vi "GetParameterValueBoolean.vi"(8 "error in (no error)":errorcluster, 11 "Parameter in":refnum<class "Parameter.lvclass">) -> (0 "error out":errorcluster, 2 "Value":bool, 3 "Parameter out":refnum<class "Parameter.lvclass">)   [LabVIEW 2023, in "Easy.SequenceManagerLabVIEW.lvlib" / "Parameter.lvclass"]
uses:
  Parameter.lvclass
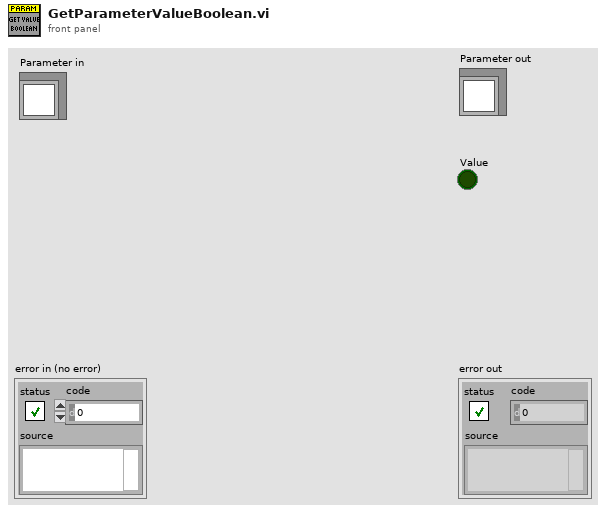
[diagram p1: front panel]
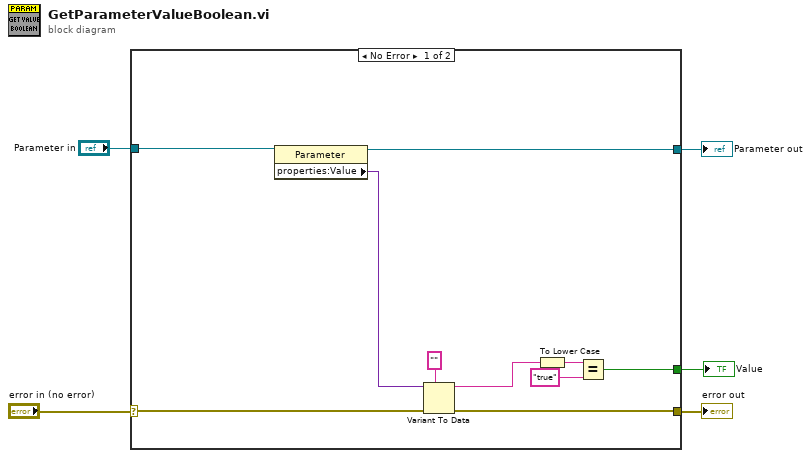
[diagram p0: block diagram]
diagram:
  n1 = case shown="No Error" "error in (no error)" {
    selector: "error in (no error)" -> [w15 w17]
    tunnel: [w12 w17] -> w4
    tunnel: "Parameter in" -> [w10 w16]
    tunnel: [w11 w16] -> w2
    tunnel: [w6 _] -> w1
    frame No Error {
      n2 = property class="Parameter"(reference=w10) -> (reference out=w11:refnum<class "Parameter.lvclass">, "properties:Value"=w13:variant)  [unwired: 1 in, 1 out]
      n3 = Variant To Data(error in=w15, type="", Variant=w13) -> (data=w9:string, error out=w12:errorcluster)
      n4 = To Lower Case(string=w9) -> (all lower case string=w8:string)
      n5 = Equal?(x=w8, y="true") -> (x = y?=w6:bool)
    }
    frame Error {
    }
  }
  "error out" <- w4
  "Parameter out" <- w2
  "Value" <- w1
